vi "Close RFSA.vi"(8 "error in":errorcluster {"code" format="%.0x"}, 11 "instrument handle":refnum<k15>) -> (0 "error out":errorcluster {"code" format="%.0x"})   [LabVIEW 2018]
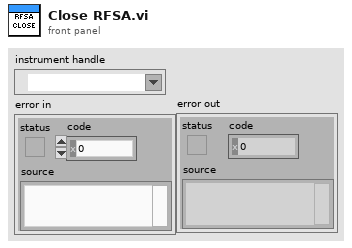
[diagram p1: front panel]
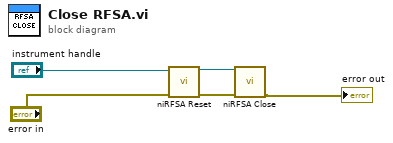
[diagram p0: block diagram]
diagram:
  n1 = call <instrlib>:"niRFSA Reset.vi"("instrument handle"="instrument handle", "error in"="error in") -> ("instrument handle out"=w3:refnum<k15>, "error out"=w2:errorcluster)  [unwired: 12 in]
  n2 = call <instrlib>:"niRFSA Close.vi"("instrument handle"=w3, "error in"=w2) -> ("error out"=→"error out":errorcluster)  [unwired: 13 in]
